vi "for_condicional_vi.vi"() -> ()   [LabVIEW 2020]
panel:
  out "Array 2":dbl[](array[numeric])
  out "Array":i32[](array[numeric])
  out "Thermometer":dbl(slide) scale=0.0..100.0
  out "Iteraciones":i32
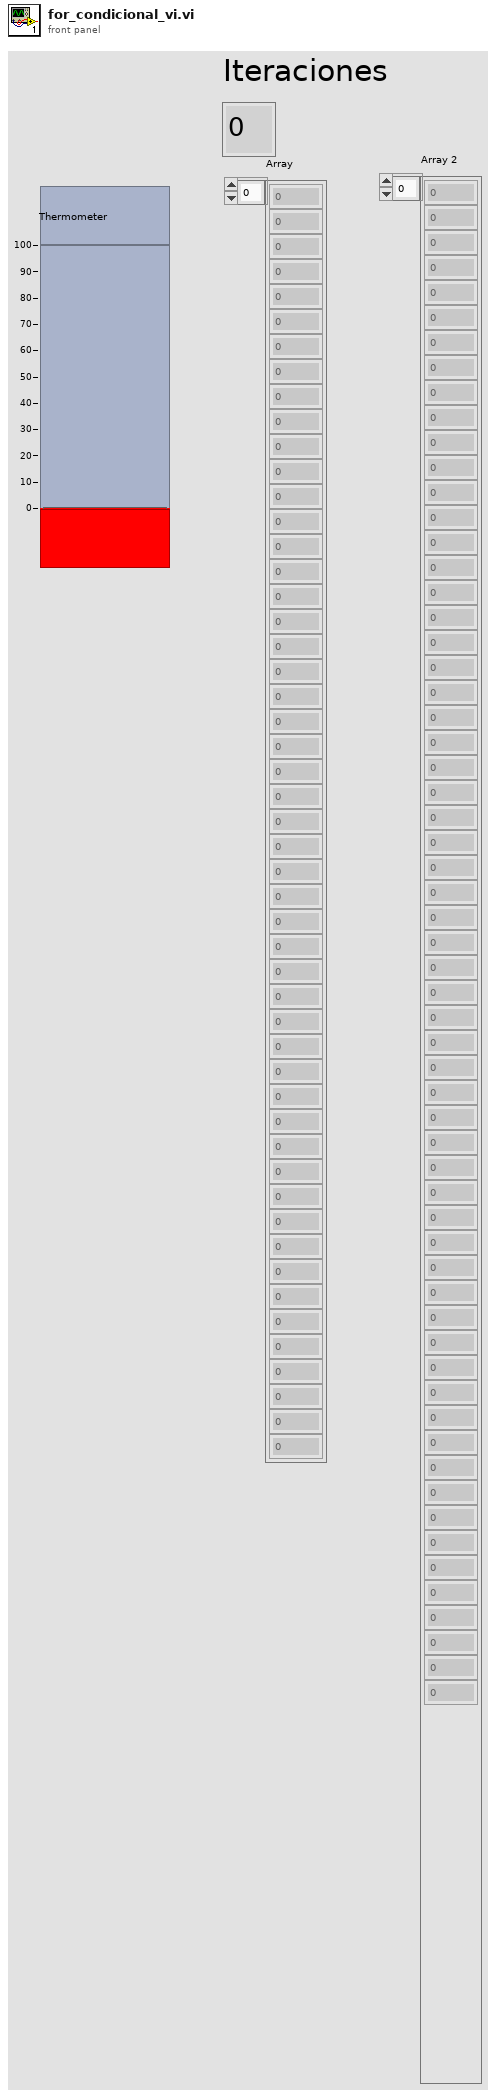
[diagram p1: front panel]
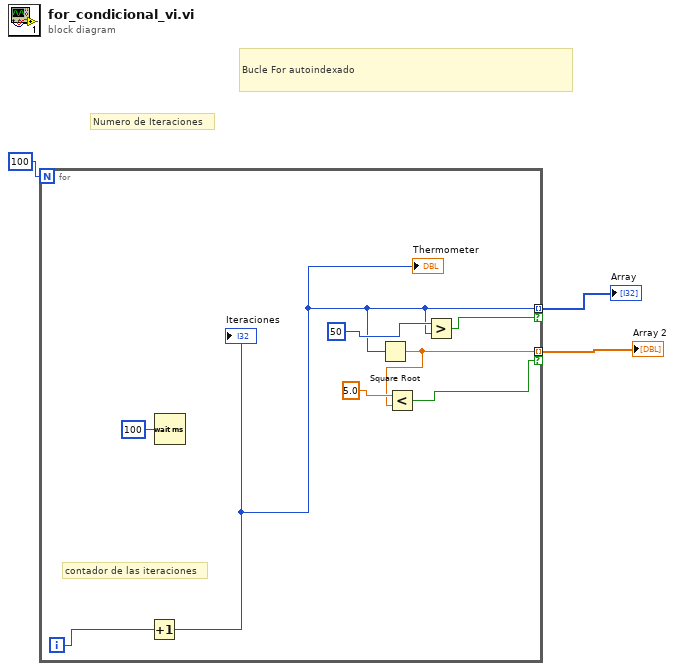
[diagram p0: block diagram]
diagram:
  # "Bucle For autoindexado"
  # "Numero de Iteraciones"
  n1 = for {
    N: 100 -> [_]
    tunnel: [w8] -> w2 mode=indexing if=w7
    tunnel: [w4] -> w1 mode=indexing if=w6
    i -> [w10]
    # "contador de las iteraciones"
    n2 = Increment(x=w10) -> (x+1=w8:i32)
    "Iteraciones" <- w8
    "Thermometer" <- w8
    n3 = Wait (ms)(milliseconds to wait=u32 100) -> ()  [unwired: 1 out]
    n4 = Square Root(x=w8) -> (sqrt(x)=w4:dbl)
    n5 = Less?(x=5.0, y=w4) -> (x < y?=w6:bool)
    n6 = Greater?(x=50, y=w8) -> (0:w7:bool)
  }
  "Array" <- w2
  "Array 2" <- w1
